vi "Excel_Insert_Panel.vi"(0 "Worksheet":refnum<k7>, 1 "Excel.Shapes":refnum<k7>, 5 "VI name":string, 7 "image file type(.jpg)":enum16{".jpg", ".png"}(ring), 9 "visible area only":bool, 11 "error in (no error)":errorcluster, 12 "Image depth":u16(ring)=3 items=["B&W", "4 bits", "8 bits", "24 bits"], 13 "name":string, 14 "Position (Excel)":cluster{"row":i32, "column":i32}) -> (15 "error out":errorcluster)   [LabVIEW 2010, in "NI_ReportGenerationToolkit.lvlib"]
uses:
  <vilib>/addons/_office/NI_ReportGenerationToolkit.lvlib
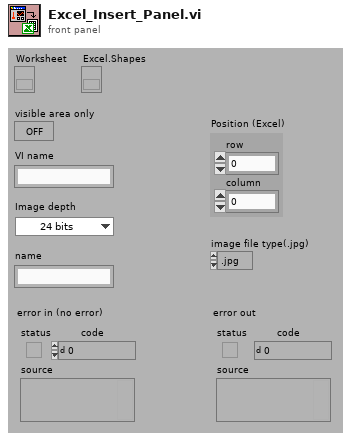
[diagram p1: front panel]
types:
  T1 = typedef "imagedata.ctl" = cluster{"image type":i32, "image depth":i32, "image":u8[], "mask":u8[], "colors":u32[], "Rectangle":cluster{"left":i16, "top":i16, "right":i16, "bottom":i16}}
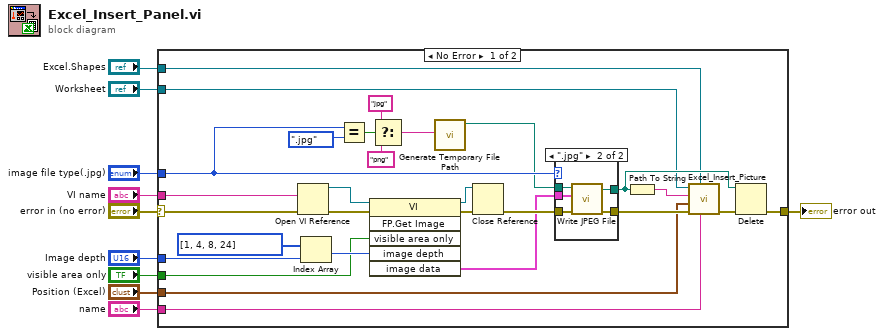
[diagram p0: block diagram]
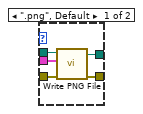
[diagram p2: hidden frame]
diagram:
  n1 = case shown="No Error" "error in (no error)" {
    selector: "error in (no error)" -> [w25 w49]
    tunnel: "VI name" -> [w38 _]
    tunnel: "Image depth" -> [w36 _]
    tunnel: [w35 w49] -> w8
    tunnel: "Excel.Shapes" -> [w23 _]
    tunnel: "image file type(.jpg)" -> [w17 _]
    tunnel: "visible area only" -> [w15 _]
    tunnel: "Worksheet" -> [w14 _]
    tunnel: "Position (Excel)" -> [w13 _]
    tunnel: "name" -> [w12 _]
    frame No Error {
      n2 = Open VI Reference(vi path=w38, error in (no error)=w25) -> (vi reference=w34:refnum<vi>, error out=w33:errorcluster)  [unwired: 4 out]
      n3 = Index Array(array=i32[] [1, 4, 8, 24] ("Array Constant"), index=w36) -> (element=w24:i32)
      n4 = Equal?(x=w17, y=enum16{".jpg", ".png"}.".jpg") -> (x = y?=w21:bool)
      n5 = invoke class="VI" method="FP.Get Image"(reference=w34, error in=w33, "visible area only"=w15, "image depth"=w24) -> (reference out=w28:refnum<vi>, error out=w27:errorcluster, "image data"=w11:T1)  [unwired: 2 in, 3 out]
      n6 = Select(t="jpg", s=w21, f="png") -> (s? t:f=w20:string)
      n7 = call <vilib>:"Generate Temporary File Path.vi"("Temporary File Extension (tmp)"=w20) -> ("Unique Temporary File Path"=w16:path)  [unwired: 1 in, 9 out]
      n8 = Close Reference(reference=w28, error in (no error)=w27) -> (error out=w26:errorcluster)
      n9 = case shown="\".jpg\"" w17 {
        tunnel: w11 -> [w39 w44]
        tunnel: w16 -> [w43 w48]
        tunnel: w26 -> [w42 w47]
        tunnel: [w41 w46] -> w30
        tunnel: [w40 w45] -> w32
        frame ".png", Default {
          n10 = call <vilib>:"Write PNG File.vi"("error in (no error)"=w42, "image data"=w39, "path to PNG file"=w43) -> ("error out"=w41:errorcluster, "path"=w40:path)  [unwired: 1 in, 6 out]
        }
        frame ".jpg" {
          n11 = call <vilib>:"Write JPEG File.vi"("error in (no error)"=w47, "image data"=w44, "path to JPEG file"=w48) -> ("error out"=w46:errorcluster, "path"=w45:path)  [unwired: 7 out]
        }
      }
      n12 = Path To String(path=w32) -> (string=w31:string)
      n13 = call <vilib>:"Excel_Insert_Picture.vi"("name"=w12, "Shapes"=w23, "error in (no error)"=w30, "position"=w13, "Filename"=w31, "Worksheet"=w14) -> ("error out"=w29:errorcluster)  [unwired: 5 out]
      n14 = Delete(path (use dialog)=w32, error in=w29) -> (error out=w35:errorcluster)  [unwired: 5 out]
    }
    frame Error {
    }
  }
  "error out" <- w8
